vi "Sandbox.vi"(8 "error in (no error)":errorcluster, 11 "VIPM in":refnum<class "VIPM.lvclass">) -> (0 "error out":errorcluster, 3 "VIPM out":refnum<class "VIPM.lvclass">)   [LabVIEW 2019, in "VIPM.lvclass"]
uses:
  VIPM.lvclass
  VIPM.lvclass/VIPM.ctl
  <vilib>/JKI/VIPM API/VIPM API_vipm_api.lvlib
panel:
  out "Build Spec Summary":string="AH2500A 1.1.1.5\n\nProduct Description:\nLabVIEW drivers for Andeen-Hagerling 2500A capacitance bridge\n\nRelease Notes:\n[1.1.1]\n- Update to LV2019 and Instrument Framework v1.11.0\n\n---\n\nKrohn-Hite 7008 Drivers 1.7.3.33\n\nProduct Description:\nDrivers and control interface for Krohn-Hite 7008 multichannel amplifiers.\n\nRelease Notes:\n[1.7.3]\n- Update to Instrument Framework v1.11.0\n\n---\n\nLEIDEN TC 1.0.2.7\n\nProduct Description:\nTools used by LevyLab to interact with Leiden Temperature Control (TC)\n\n[Instrument.TC.MNK.lvclass]\n[Instrument.TC.CF.lvclass]\n- APIs that overrides \"Get Temperature.vi\" method of Instrument.Cryostat.lvclass\n\nRelease Notes:\n[1.0.2]\n- Fix CF Read T\n\n---\n\nCryostation 1.2.3.7\n\nProduct Description:\nProgram for logging Montana Instruments Cryostation status to the SQL DB. Provides a UI and API for getting information from the Cryostation.\n\nRelease Notes:\n[1.2.3]\n- Update to Instrument Framework v1.11.0\n\n---\n\nOxford-1820 1.3.3.23\n\nProduct Description:\nVIs for controlling the Oxford 18/20 magnet\n\nRelease Notes:\n- update to Instrument Framework v1.13.0\n\n---\n\nOxford-VRM 21.6.2.8\n\nProduct Description:\nVIs for controlling the Oxford VRM PS that controls the CF900's 3D magnet\n\nRelease Notes:\n[21.6.1]\n- Update to Instrument Framework v1.11.1\n\n---\n\nPPMS Monitor and Control 1.8.4.56\n\nProduct Description:\n- Log instrument status to the PGSQL database.\n- UI and API for controlling magnet field, temperature, and rotator angle (PPM2 only)\n\nRelease Notes:\n[1.8.4]\n- Update to Instrument Framework v1.11.1.15 (and SMO v1.4.0.69)\n- Fix Set methods\n\n---\n\nRazorbill RP100 21.2.3.9\n\nProduct Description:\nDivers for Razorbill RP100 HV amplifier\n\nRelease Notes:\n[21.2.4]\n- Update to  IF 1.11.1.15\n\n---\n"
  out "Path":path=path "C:/Users/patrick/Documents/GitHub/Razorbill-RP100/build support/Razorbill RP100.vipb"
  in  "Paths":path[](array[path])=[path "C:/Users/patrick/Documents/GitHub/Andeen-Hagerling-2500A/build support/AH2500A.vipb", path "C:/Users/patrick/Documents/GitHub/Krohn-Hite-7008/build support/Krohn Hite 7008.vipb", path "C:/Users/patrick/Documents/GitHub/Leiden-MNK-TC/build support/LEIDEN TC.vipb", path "C:/Users/patrick/Documents/GitHub/Montana-Instruments-Cryostation/build support/Cryostation.vipb", path "C:/Users/patrick/Documents/GitHub/Oxford-1820/build support/Oxford 1820 API.vipb", path "C:/Users/patrick/Documents/GitHub/Oxford-VRM/build support/Oxford VRM API.vipb", path "C:/Users/patrick/Documents/GitHub/PPMS-Monitor-and-Control/build support/PPMS Instrument.vipb", path "C:/Users/patrick/Documents/GitHub/Razorbill-RP100/build support/Razorbill RP100.vipb"]
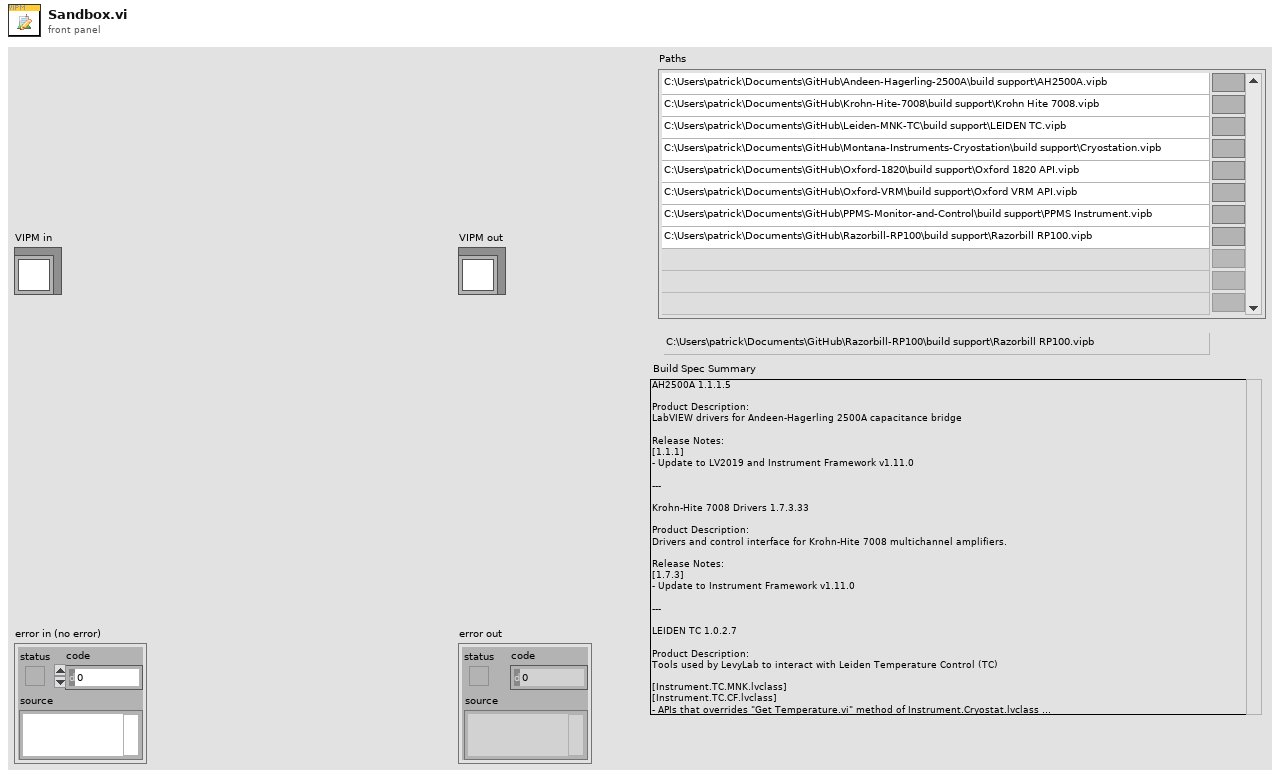
[diagram p1: front panel]
types:
  T1 = typedef "VIPM API_vipm_api.lvlib/VI Package Build Spec Data Cluster_vipm_api.ctl" = cluster{"Package Version":T2, "Product Name":string, "Company Name":string, "Author Name (Person or Company)":string, "Product Homepage (URL)":string, "Legal Copyright":string, "License Agreement Name":string, "Product Description Summary":string, "Product Description":string, "Release Notes - Change Log":string}
  T2 = typedef "VIPM API_vipm_api.lvlib/Version Info Cluster_vipm_api.ctl" = cluster{"major":u32, "minor":u32, "patch":u32, "build":u32}
  T3 = typedef "VIPM API_vipm_api.lvlib/Repository Info Cluster_vipm_api.ctl" = cluster{"Repository Name":string, "Repository Folder Location":path}
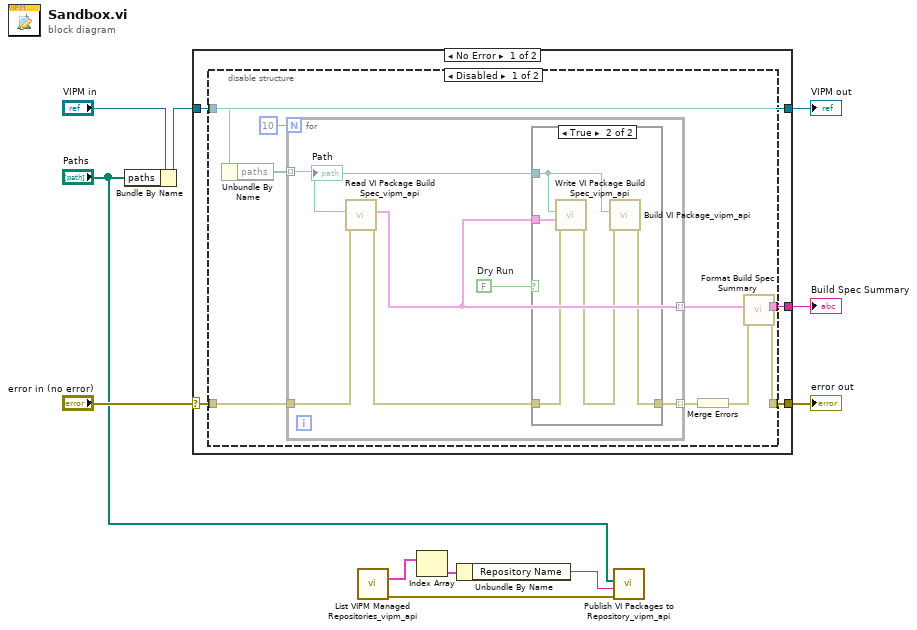
[diagram p0: block diagram]
diagram:
  n1 = Bundle By Name(cluster="VIPM in", "paths"="Paths") -> (w7:refnum<class "VIPM.lvclass">)
  n2 = case shown="No Error" "error in (no error)" {
    selector: "error in (no error)" -> [w14 w38]
    tunnel: [w12 w38] -> w10
    tunnel: [w15 w37] -> w9
    tunnel: w7 -> [w15 w37]
    tunnel: [w13 _] -> w6
    frame No Error {
      n3 = disable-structure shown="Disabled" {
        disable-tunnel: w15 -> [w24 _]
        disable-tunnel: w14 -> [w22 _]
        disable-tunnel: [w18 _] -> w13
        disable-tunnel: [w16 _] -> w12
        frame Disabled {
          n4 = Unbundle By Name(w24) -> ("paths"=w23:path[])
          n5 = for {
            N: 10 -> [_]
            tunnel: w23 -> [w26] mode=indexing
            tunnel: w22 -> [w30]
            tunnel: [w28] -> w21 mode=indexing
            tunnel: [w25] -> w19 mode=indexing
            w27 = FALSE  # Dry Run
            n6 = call <vilib>:"Read VI Package Build Spec_vipm_api.vi"("error in (no error)"=w30, "Path to VIPB File"=w26) -> ("error out"=w29:errorcluster, "VI Package Build Spec Data"=w25:T1)  [unwired: 8 in]
            n7 = case shown="True" w27 {
              tunnel: w26 -> [_ w32]
              tunnel: w29 -> [w31 w36]
              tunnel: [w31 w35] -> w28
              tunnel: w25 -> [_ w33]
              frame False {
              }
              frame True {
                n8 = call <vilib>:"Write VI Package Build Spec_vipm_api.vi"("error in (no error)"=w36, "VI Package Build Spec Data"=w33, "Path to VIPB File"=w32) -> ("error out"=w34:errorcluster)  [unwired: 8 in]
                n9 = call <vilib>:"Build VI Package_vipm_api.vi"("error in (no error)"=w34, "Path to VIPB File"=w32) -> ("error out"=w35:errorcluster)  [unwired: 8 in, 1 out]
              }
            }
            "Path" <- w26
          }
          n10 = Merge Errors(w21) -> (w17:errorcluster)
          n11 = call "Format Build Spec Summary.vi"("error in (no error)"=w17, "Build Spec [] in"=w19) -> ("error out"=w16:errorcluster, "VIPB Preview"=w18:string)  [unwired: 8 in]
        }
        frame Enabled {
        }
      }
    }
    frame Error {
    }
  }
  "error out" <- w10
  "VIPM out" <- w9
  "Build Spec Summary" <- w6
  n12 = call <vilib>:"List VIPM Managed Repositories_vipm_api.vi"() -> ("Managed Repositories Info"=w2:T3[], "error out"=w3:errorcluster)  [unwired: 14 in]
  n13 = Index Array(array=w2) -> (element=w4:T3)  [unwired: 1 in]
  n14 = Unbundle By Name(w4) -> ("Repository Name"=w5:string)
  n15 = call <vilib>:"Publish VI Packages to Repository_vipm_api.vi"("error in (no error)"=w3, "Repository Name"=w5, "Packages to publish to Repository Library (vip,ogp)"="Paths") -> ()  [unwired: 7 in, 2 out]
